vi "Add Point.vi"(0 "Data3D in":refnum<class "Data3D.lvclass">, 5 "Inner Loop":T2, 7 "Outer Loop":T1, 9 "Z":dbl, 11 "error in (no error)":errorcluster) -> (4 "Data3D out":refnum<class "Data3D.lvclass">, 15 "error out":errorcluster)   [LabVIEW 2014, in "Data3D.lvclass"]
uses:
  Data3D.lvclass
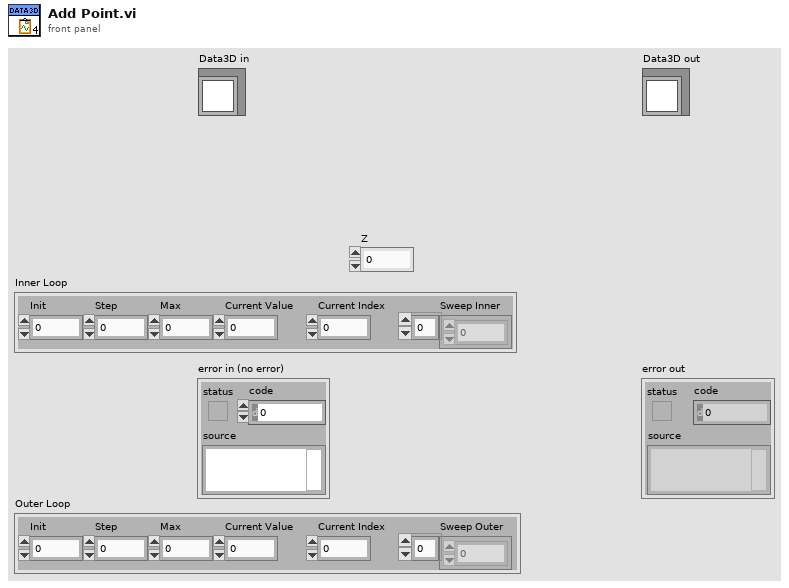
[diagram p1: front panel]
types:
  T1 = cluster{"Init":dbl, "Step":dbl, "Max":dbl, "Current Value":dbl, "Current Index":dbl, "Sweep Outer":dbl[]}
  T2 = cluster{"Init":dbl, "Step":dbl, "Max":dbl, "Current Value":dbl, "Current Index":dbl, "Sweep Inner":dbl[]}
  T3 = typedef "NI_Matrix.lvlib/RealMatrix.ctl" = dbl[][]
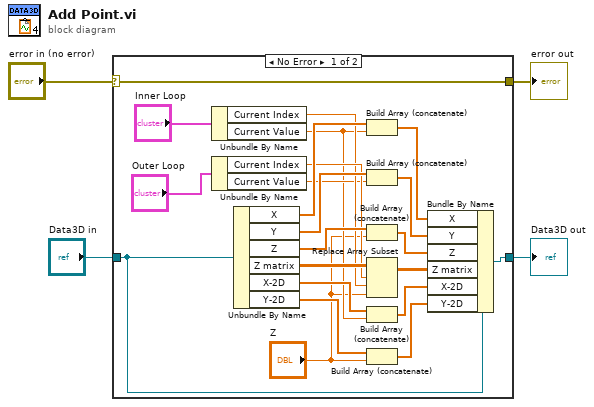
[diagram p0: block diagram]
diagram:
  n1 = case shown="No Error" "error in (no error)" {
    selector: "error in (no error)" -> [w26 w28]
    tunnel: [w26 w28] -> w3
    tunnel: [w21 w27] -> w1
    tunnel: "Data3D in" -> [w22 w27]
    frame No Error {
      n2 = Unbundle By Name("Inner Loop") -> ("Current Index"=w13:dbl, "Current Value"=w8:dbl)
      n3 = Unbundle By Name("Outer Loop") -> ("Current Index"=w14:dbl, "Current Value"=w11:dbl)
      n4 = Unbundle By Name(w22) -> ("X"=w25:dbl[], "Y"=w24:dbl[], "Z"=w23:dbl[], "Z matrix"=w15:dbl[][], "X-2D"=w10:dbl[], "Y-2D"=w7:dbl[])
      n5 = Build Array (concatenate)(w25, w8) -> (w20:dbl[])
      n6 = Build Array (concatenate)(w24, w11) -> (w19:dbl[])
      n7 = Build Array (concatenate)(w23, "Z") -> (w18:dbl[])
      n8 = Replace Array Subset(array=w15, new element="Z", index (row)=w14, index (col)=w13) -> (w12:T3)
      n9 = Build Array (concatenate)(w10, w8) -> (w9:dbl[])
      n10 = Build Array (concatenate)(w7, "Z") -> (w5:dbl[])
      n11 = Bundle By Name(cluster=w22, "X"=w20, "Y"=w19, "Z"=w18, "Z matrix"=w12, "X-2D"=w9, "Y-2D"=w5) -> (w21:refnum<class "Data3D.lvclass">)
    }
    frame Error {
    }
  }
  "error out" <- w3
  "Data3D out" <- w1
